vi "ScanSteuerung_to_DSPText.vi"(1 "ScanSteuerungOut":T1) -> (0 "String":string="AV,0,3,-1361800\r\nAV,0,4,-2540500\r\nAV,0,5,0\r\nAI,0,3,1315\r\nAI,0,4,0\r\nAI,0,5,0\r\nAS,120,9,751\r\nAV,120,1,2\r\nAI,3134,3,-45281\r\nAI,3134,4,60\r\nAI,3134,5,1\r\nAI,3225,3,1315\r\nAI,3225,4,0\r\nAI,3225,5,0\r\nAV,3254,1,3\r\nAE,3345,9,0\r\nAV,2422095,1,2\r\nAI,2425108,3,0\r\nAI,2425108,4,0\r\nAI,2425108,5,0\r\nAV,2425228,1,0\r\n")   [LabVIEW 2011]
uses:
  ScanControl.ctl
  ScanControl_Action.ctl
  ScanControl_Channel.ctl
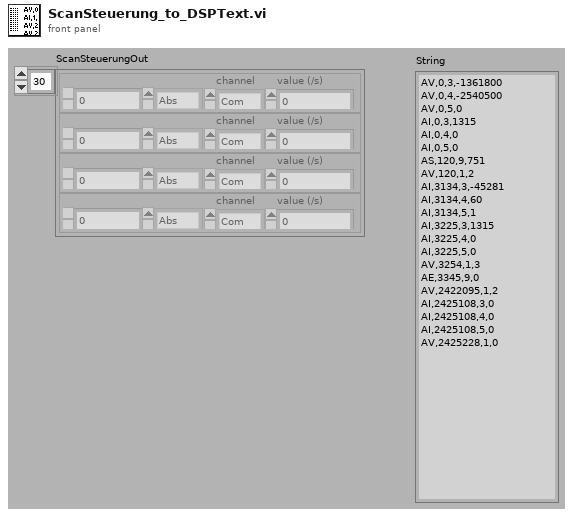
[diagram p1: front panel]
types:
  T1 = typedef "ScanControl.ctl" = cluster{"Time [s]":dbl, "action":T2, "channel":T3, "value (/s)":dbl}[]
  T2 = typedef "ScanControl_Action.ctl" = enum16{"Abs", "Rel", "Inc", "IncInc", "LoopStart", "LoopEnd", "WaitTriggerRising"}
  T3 = typedef "ScanControl_Channel.ctl" = enum16{"Com", "AnalogConfig", "AnalogValue", "GalvoX", "GalvoY", "Galvo3", "Galvo4", "Digital", "Free", "Loop", "SMoveTime", "Image1X", "Image1Y", "Image2X", "Image2Y"}
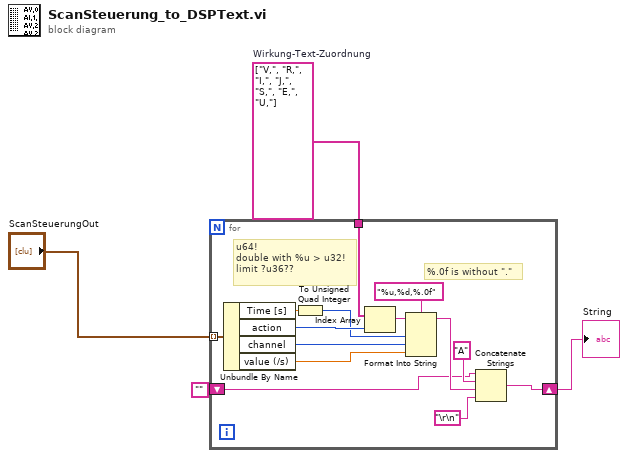
[diagram p0: block diagram]
diagram:
  w1 = string[] ["V,", "R,", "I,", "J,", "S,", "E,", "U,"]  # Wirkung-Text-Zuordnung
  n1 = for {
    tunnel: "ScanSteuerungOut" -> [w5] mode=indexing
    tunnel: w1 -> [w16]
    shift-right: [w17] -> w2
    shift-left: "" -> [w9]
    # "u64!\ndouble with %u > u32!\nlimit ?u36??"
    # "%.0f is without \".\""
    n2 = Unbundle By Name(w5) -> ("Time [s]"=w7:dbl, "action"=w15:T2, "channel"=w12:T3, "value (/s)"=w8:dbl)
    n3 = To Unsigned Quad Integer(1:w7) -> (0:w6:u64)
    n4 = Index Array(array=w16, index=w15) -> (element=w14:string)
    n5 = Format Into String(format string="%u,%d,%.0f" ("Format String"), initial string=w14, w6, w12, w8) -> (resulting string=w11:string)  [unwired: 1 in, 1 out]
    n6 = Concatenate Strings(w9, "A", w11, "\r\n") -> (w17:string)
  }
  "String" <- w2
